vi "MainTester.vi"() -> ()   [LabVIEW 2015]
uses:
  <vilib>/Rock Robotics/WPI/SerialPort/WPI_SerialPortRef.ctl
  <vilib>/Rock Robotics/WPI/SerialPort/WPI_SerialPort.ctl
panel:
  out "ADC voltages":dbl[](array[numeric])
  out "error out 4":errorcluster
  out "SerialPortRef 3":T1
  out "error out 3":errorcluster
  out "SerialPortRef 2":T1
  out "error out 2":errorcluster
  out "All Digital Input Vals":bool[](array[boolean])
  out "error out":errorcluster
  in  "stop":bool
  in  "error in (no error)":errorcluster
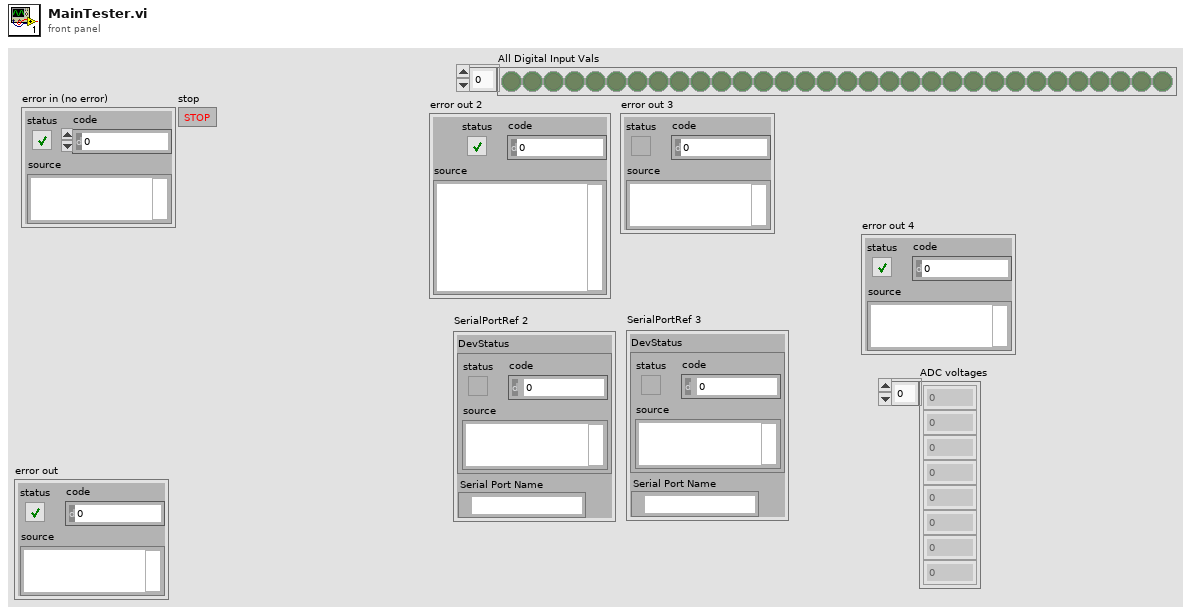
[diagram p1: front panel]
types:
  T1 = typedef "WPI_SerialPortRef.ctl" = cluster{"DevStatus":errorcluster, "Serial Port Name":refnum<visa-resource-name>}
  T2 = typedef "WPI_SerialPort.ctl" = enum16{"Onboard RS-232", "MXP TTL"}
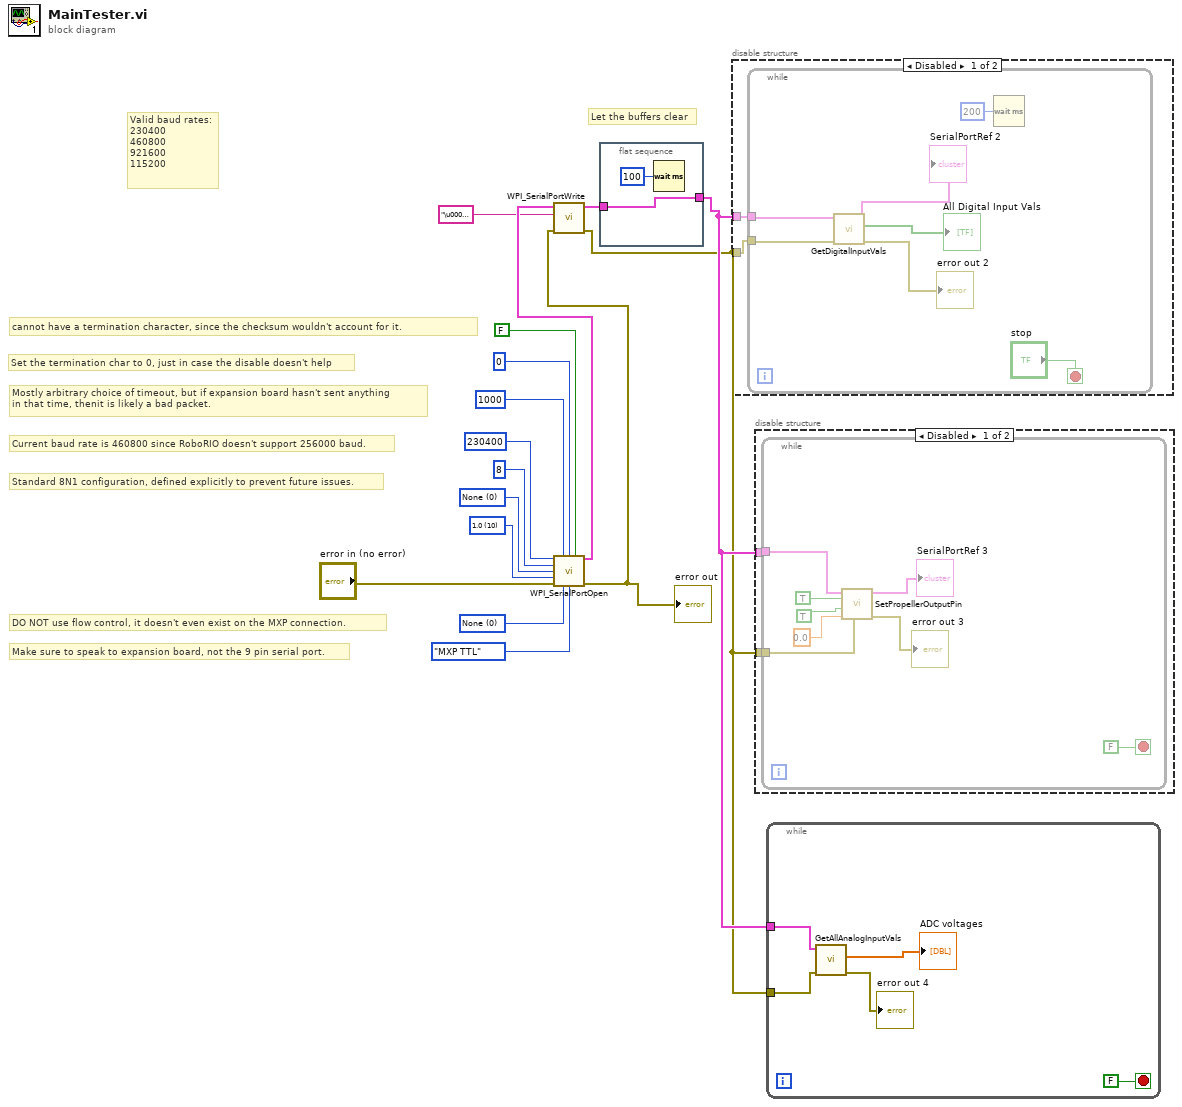
[diagram p0: block diagram]
diagram:
  w15 = u16 10 items=["1.0"=10, "1.5"=15, "2.0"=20] ("Stop Bits")
  w11 = u16 0 items=["None", "XON/XOFF", "RTS/CTS", "XON/XOFF & RTS/CTS", "DTR/DSR", "XON/XOFF & DTR/DSR"] ("Flow Control")
  w10 = u16 0 items=["None", "Odd", "Even", "Mark", "Space"] ("Parity")
  # "Let the buffers clear"
  # "Valid baud rates:\n230400\n460800\n921600\n115200"
  # "Make sure to speak to expansion board, not the 9 pin serial port."
  # "DO NOT use flow control, it doesn't even exist on the MXP connection."
  # "Standard 8N1 configuration, defined explicitly to prevent future issues."
  # "Current baud rate is 460800 since RoboRIO doesn't support 256000 baud."
  # "Mostly arbitrary choice of timeout, but if expansion board hasn't sent anything\nin that time, thenit is likely a bad packet."
  # "Set the termination char to 0, just in case the disable doesn't help"
  # "cannot have a termination character, since the checksum wouldn't account for it."
  n1 = call <vilib>:"WPI_SerialPortOpen.vi"("Baud Rate"=u32 230400, "Timeout Value (ms)"=u32 1000, "Termination Char (0xA = '\\n' = LF)"=u8 0 ("Termination Char (0xA = '\\n' = LF)"), "Enable Termination Char? (T)"=FALSE, "Data Bits"=u16 8, "Parity"=w10, "Stop Bits"=w15, "error in (no error)"="error in (no error)", "Flow Control"=w11, "Serial Port"=WPI_SerialPort."MXP TTL") -> ("SerialPortRef"=w6:T1, "error out"=w5:errorcluster)  [unwired: 4 in]
  "error out" <- w5
  n2 = call <vilib>:"WPI_SerialPortWrite.vi"("error in (no error)"=w5, "Buffer"="\u0004\u0004", "SerialPortRef"=w6) -> ("error out"=w1:errorcluster, "SerialPortRef"=w3:T1)  [unwired: 6 in, 1 out]
  n3 = flat-sequence {
    tunnel: [w18] -> w2
    tunnel: w3 -> [w18]
    frame #0 {
      n4 = Wait (ms)(milliseconds to wait=u32 100) -> ()  [unwired: 1 out]
    }
  }
  n5 = disable-structure shown="Disabled" {
    disable-tunnel: w1 -> [w20 _]
    disable-tunnel: w2 -> [w19 _]
    frame Disabled {
      n6 = while {
        tunnel: w20 -> [w25]
        tunnel: w19 -> [w26]
        stop <- "stop" stop-if-true
        n7 = call "GetDigitalInputVals.vi"("error in (no error)"=w25, "SerialPortRef"=w26) -> ("error out"=→"error out 2":errorcluster, "All Digital Input Vals"=→"All Digital Input Vals":bool[], "SerialPortRef 2"=→"SerialPortRef 2":T1)  [unwired: 7 in]
        n8 = Wait (ms)(milliseconds to wait=u32 200) -> ()  [unwired: 1 out]
      }
    }
    frame Enabled {
    }
  }
  n9 = disable-structure shown="Disabled" {
    disable-tunnel: w1 -> [w29 _]
    disable-tunnel: w2 -> [w28 _]
    frame Disabled {
      n10 = while {
        tunnel: w29 -> [w34]
        tunnel: w28 -> [w31]
        stop <- FALSE stop-if-true
        n11 = call "SetPropellerOutputPin.vi"("error in (no error)"=w34, "Pin Number"=0.0, "Value"=TRUE, "Dir"=TRUE, "SerialPortRef"=w31) -> ("error out"=→"error out 3":errorcluster, "SerialPortRef 2"=→"SerialPortRef 3":T1)  [unwired: 5 in]
      }
    }
    frame Enabled {
    }
  }
  n12 = while {
    tunnel: w2 -> [w42]
    tunnel: w1 -> [w41]
    stop <- FALSE stop-if-true
    n13 = call "GetAllAnalogInputVals.vi"("error in (no error)"=w41, "SerialPortRef"=w42) -> ("error out"=→"error out 4":errorcluster, "ADC voltages"=→"ADC voltages":dbl[])  [unwired: 6 in, 2 out]
  }
